vi "NoParent_TagNameIncludesPrefixAndName.vi"() -> (0 "error out":errorcluster)   [LabVIEW 2017, in "ResultTree.Tests.lvlib" / "AddTestCase.lvlib"]
uses:
  AddTestCase.lvlib
  c09b0184-a7a5-4658-999a-d2ef6d2e958d.vi
  Constraint/IsEqual/Create.vi
  Constraint/IsEqual/IsEqual.lvclass
  ResultTree/ResultTree.lvclass
panel:
  in  "Tree":string(tree)
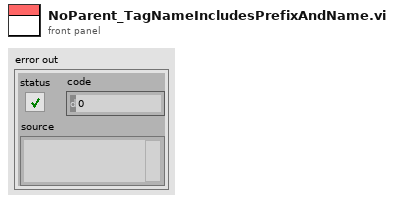
[diagram p1: front panel]
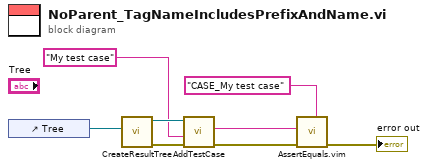
[diagram p0: block diagram]
diagram:
  n1 = control-ref of="Tree"() -> (w7:refnum<vi>)
  n2 = call "CreateResultTree.vi"("Tree Refnum"=w7) -> ("error out"=w6:errorcluster, "ResultTree out"=w4:refnum<class "ResultTree.lvclass">)  [unwired: 9 in]
  n3 = call "AddTestCase.vi"("error in (no error)"=w6, "Name"="My test case", "ResultTree in"=w4) -> ("error out"=w5:errorcluster, "Tag"=w1:string)  [unwired: 6 in, 1 out]
  n4 = call "AssertEquals.vim"("Expected"="CASE_My test case" ("Name"), "error in (no error)"=w5, "Actual"=w1) -> ("error out"=→"error out":errorcluster)  [unwired: 8 in]
